vi "TS Run Stop.vi"(8 "error in (no error)":errorcluster, 11 "HTS Test Stand in":refnum<class "HTS Test Stand.lvclass">) -> (0 "error out":errorcluster, 3 "HTS Test Stand out":refnum<class "HTS Test Stand.lvclass">)   [LabVIEW 2019, in "Test Stands.lvlib" / "HTS Test Stand.lvclass"]
uses:
  HTS Test Stand.lvclass
  Results/Results Method.ctl
  Results/Results.lvlib
  Results/HTS Results/HTS Results.lvclass
  C:/Users/wg/Documents/LV_Projects/test-stand/App/Results/Results.lvclass
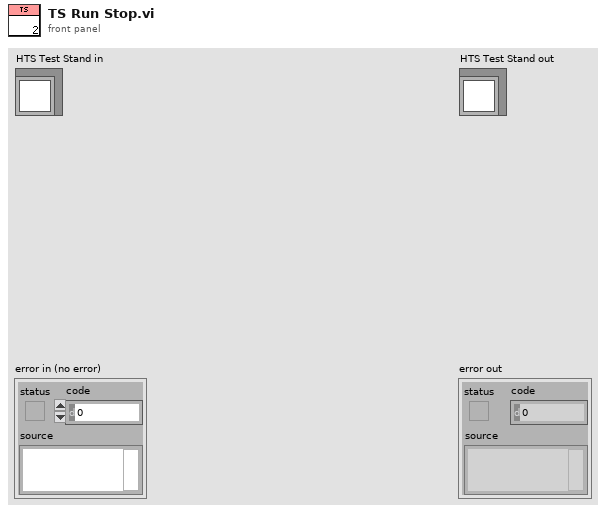
[diagram p1: front panel]
types:
  T1 = typedef "Results.lvlib/Results Method.ctl" = enum16{"Get", "Set"}
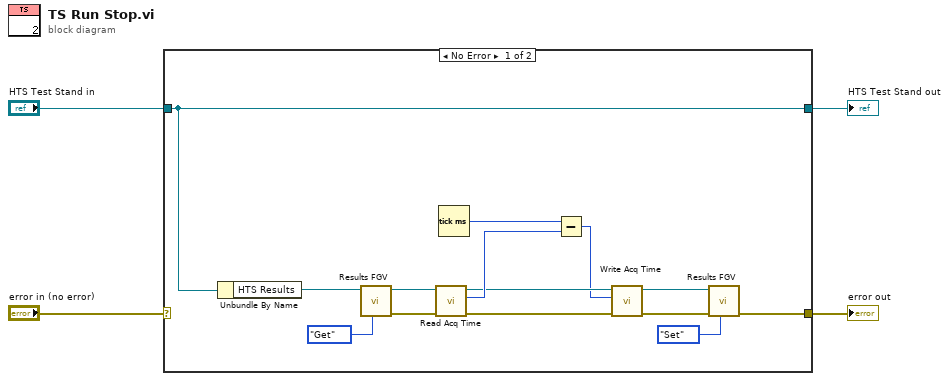
[diagram p0: block diagram]
diagram:
  n1 = case shown="No Error" "error in (no error)" {
    selector: "error in (no error)" -> [_ w20]
    tunnel: [w5 w20] -> w1
    tunnel: [w9 w19] -> w2
    tunnel: "HTS Test Stand in" -> [w9 w19]
    frame No Error {
      n2 = Unbundle By Name(w9) -> ("HTS Results"=w17:refnum<class "HTS Results.lvclass">)
      n3 = call-dynamic "Results FGV.vi"("Method"=Results_Method."Get", "HTS Results in"=w17) -> ("error out"=w14:errorcluster, "HTS Results out"=w15:refnum<class "HTS Results.lvclass">)  [unwired: 8 in]
      n4 = call "Read Acq Time.vi"("error in (no error)"=w14, "Results in"=w15) -> ("error out"=w10:errorcluster, "Acq Time"=w13:u32, "Results out"=w11:refnum<class "HTS Results.lvclass">)  [unwired: 7 in]
      n5 = Tick Count (ms)() -> (millisecond timer value=w12:u32)
      n6 = Subtract(x=w12, y=w13) -> (x-y=w6:u32)
      n7 = call "Write Acq Time.vi"("error in (no error)"=w10, "Acq Time"=w6, "Results in"=w11) -> ("error out"=w7:errorcluster, "Results out"=w8:refnum<class "HTS Results.lvclass">)  [unwired: 7 in]
      n8 = call-dynamic "Results FGV.vi"("Method"=Results_Method."Set", "error in"=w7, "HTS Results in"=w8) -> ("error out"=w5:errorcluster)  [unwired: 7 in, 1 out]
    }
    frame Error {
    }
  }
  "error out" <- w1
  "HTS Test Stand out" <- w2
